vi "Simple TCP Test.vi"() -> ()   [LabVIEW 2020, in "VectoScratch.lvlib"]
uses:
  VectoScratch.lvlib
  Vecto/TCPMessaging/TCPMessaging.lvclass
  Simple TCP Handler/Simple TCP Handler.lvclass
  Vecto/TCPMessageService/TCPMessageAPI.lvclass
  Vecto/proto/TcpClientHello/Data.ctl
  Vecto/proto/TcpClientHello/TcpClientHello.lvlib
  Vecto/SequenceCountService/SequenceCountService.lvclass
  C:/dev/lv20CE/relink/lv-vecto/Vecto/TCPConnectionHandler/TCPConnectionHandler.lvclass
  C:/dev/lv20CE/relink/lv-vecto/Vecto/TCPMessageHandler/TCPMessageHandler.lvclass
  Vecto/Connection State.ctl
  Vecto/Vecto.lvlib
panel:
  out "Server Read":i32
  out "Client Read":i32
  out "Server Send":i32
  in  "Server Stop":bool
  in  "Client Stop":bool
  out "Client Send":i32
  out "Server Error":errorcluster
  out "Client Error":errorcluster
  out "Server State":T1=enum."Disconnected"
  out "Client State":T1=enum."Disconnected"
  # "Server send counts at ~half the speed of the client."
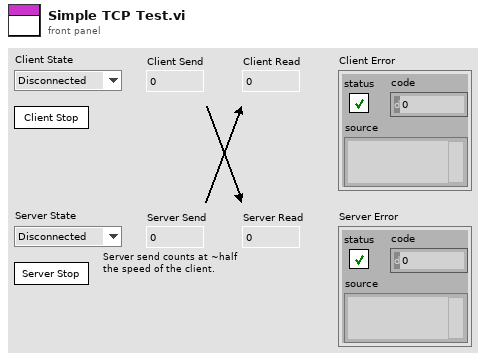
[diagram p1: front panel]
types:
  T1 = typedef "Vecto.lvlib/Connection State.ctl" = enum16{"Connected", "Disconnected"}
  T2 = typedef "TcpClientHello.lvlib/Data.ctl" = cluster{"node_id":u32, "system":string, "cluster":string, "node_name":string, "app_version":string, "config_version":string, "config_hash":string}
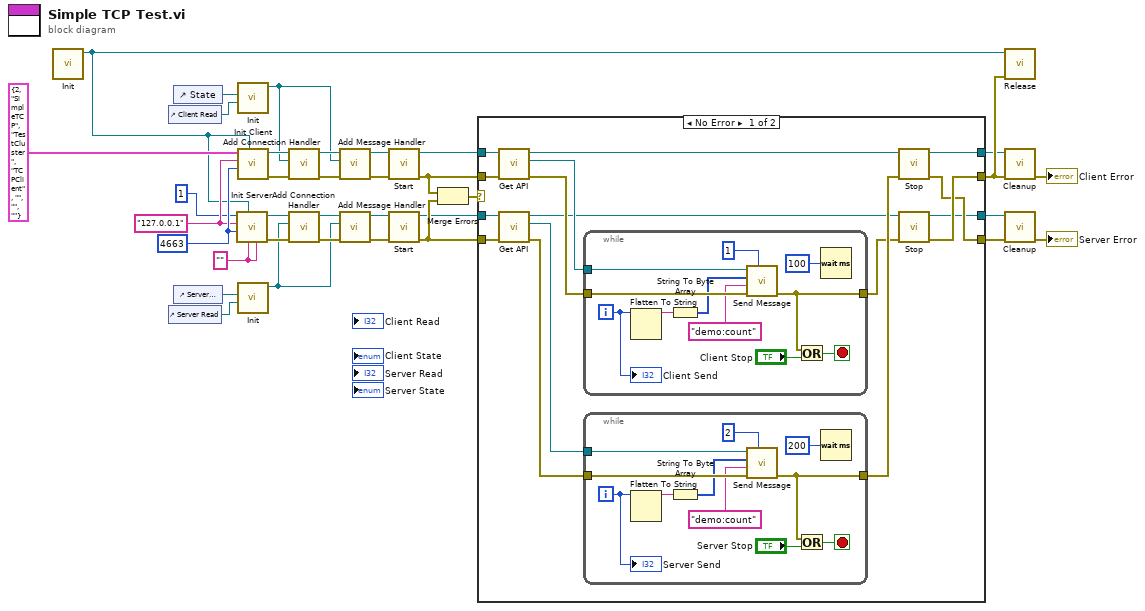
[diagram p0: block diagram]
diagram:
  w1 = "" ("Local Config Version")
  w34 = u16 4663 ("Bind Port")
  w33 = "127.0.0.1" ("Bind Address")
  n1 = call "Init.vi"() -> ("SequenceCountService out"=w2:refnum<class "SequenceCountService.lvclass">)  [unwired: 10 in, 1 out]
  n2 = control-ref of="Client Read"() -> (w5:refnum<vi>)
  n3 = control-ref of="Server Read"() -> (w6:refnum<vi>)
  n4 = control-ref of="State"() -> (w31:refnum<vi>)
  n5 = control-ref of="Server State"() -> (w23:refnum<vi>)
  n6 = call "Init Server.vi"("Local Config Hash"=w1, "Local Config Version"=w1, "SequenceCountService"=w2, "Bind Port"=w34, "Bind Address"=w33, "Node ID"=u32 1) -> ("error out"=w17:errorcluster, "TCPMessaging out"=w18:refnum<class "TCPMessaging.lvclass">)  [unwired: 4 in]
  n7 = call "Init.vi"("Value"=w5, "State"=w31) -> ("Simple TCP Handler out"=w27:refnum<class "Simple TCP Handler.lvclass">)  [unwired: 8 in, 1 out]
  n8 = call "Init Client.vi"("SequenceCountService"=w2, "Remote Port"=w34, "Remote Address"=w33, "Client Info"=T2 {"node_id"=2, "system"="SimpleTCP", "cluster"="TestCluster", "node_name"="TCPClient", "app_version"="", "config_version"="", "config_hash"=""}) -> ("error out"=w29:errorcluster, "TCPMessaging out"=w30:refnum<class "TCPMessaging.lvclass">)  [unwired: 6 in]
  n9 = call "Init.vi"("Value"=w6, "State"=w23) -> ("Simple TCP Handler out"=w4:refnum<class "Simple TCP Handler.lvclass">)  [unwired: 8 in, 1 out]
  n10 = call "Add Connection Handler.vi"("error in (no error)"=w29, "TCPConnectionHandler"=w27, "TCPMessaging in"=w30) -> ("error out"=w26:errorcluster, "TCPMessaging out"=w28:refnum<class "TCPMessaging.lvclass">)  [unwired: 7 in]
  n11 = call "Add Connection Handler.vi"("error in (no error)"=w17, "TCPConnectionHandler"=w4, "TCPMessaging in"=w18) -> ("error out"=w20:errorcluster, "TCPMessaging out"=w19:refnum<class "TCPMessaging.lvclass">)  [unwired: 7 in]
  n12 = call "Add Message Handler.vi"("error in (no error)"=w26, "TCPMessageHandler"=w27, "TCPMessaging in"=w28) -> ("error out"=w24:errorcluster, "TCPMessaging out"=w25:refnum<class "TCPMessaging.lvclass">)  [unwired: 7 in]
  n13 = call "Add Message Handler.vi"("error in (no error)"=w20, "TCPMessageHandler"=w4, "TCPMessaging in"=w19) -> ("error out"=w22:errorcluster, "TCPMessaging out"=w21:refnum<class "TCPMessaging.lvclass">)  [unwired: 7 in]
  n14 = call "Start.vi"("error in (no error)"=w24, "TCPMessaging in"=w25) -> ("error out"=w15:errorcluster, "TCPMessaging out"=w12:refnum<class "TCPMessaging.lvclass">)  [unwired: 8 in]
  n15 = call "Start.vi"("error in (no error)"=w22, "TCPMessaging in"=w21) -> ("error out"=w14:errorcluster, "TCPMessaging out"=w13:refnum<class "TCPMessaging.lvclass">)  [unwired: 8 in]
  n16 = Merge Errors(w15, w14) -> (w16:errorcluster)
  n17 = case shown="No Error" w16 {
    tunnel: w15 -> [w49 w77]
    tunnel: w14 -> [w47 w76]
    tunnel: w13 -> [w48 w75]
    tunnel: w12 -> [w50 w74]
    tunnel: [w41 w77] -> w35
    tunnel: [w39 w76] -> w9
    tunnel: [w38 w75] -> w10
    tunnel: [w40 w74] -> w11
    frame No Error {
      n18 = call "Get API.vi"("error in (no error)"=w49, "TCPMessaging in"=w50) -> ("error out"=w45:errorcluster, "TCP Messaging API"=w46:refnum<class "TCPMessageAPI.lvclass">, "TCPMessaging out"=w42:refnum<class "TCPMessaging.lvclass">)  [unwired: 7 in]
      n19 = call "Get API.vi"("error in (no error)"=w47, "TCPMessaging in"=w48) -> ("error out"=w36:errorcluster, "TCP Messaging API"=w37:refnum<class "TCPMessageAPI.lvclass">, "TCPMessaging out"=w44:refnum<class "TCPMessaging.lvclass">)  [unwired: 7 in]
      n20 = while {
        tunnel: w46 -> [w73]
        tunnel: w45 -> [w71]
        tunnel: [w64] -> w43
        i -> [w68]
        stop <- w65 stop-if-true
        n21 = Flatten To String(anything=w68) -> (data string=w70:string)  [unwired: 3 in, 2 out]
        n22 = String To Byte Array(string=w70) -> (unsigned byte array=w69:u8[])
        n23 = call "Send Message.vi"("Target ID"=u32 1 ("Target Node"), "error in (no error)"=w71, "Type"="demo:count", "Payload"=w69, "TCPMessageService in"=w73) -> ("error out"=w64:errorcluster)  [unwired: 5 in, 1 out]
        n24 = Or(x=w64, y="Client Stop") -> (x .or. y?=w65:bool)
        n25 = Wait (ms)(milliseconds to wait=u32 100) -> ()  [unwired: 1 out]
        "Client Send" <- w68
      }
      n26 = while {
        tunnel: w37 -> [w62]
        tunnel: w36 -> [w60]
        tunnel: [w53] -> w51
        i -> [w57]
        stop <- w54 stop-if-true
        n27 = Flatten To String(anything=w57) -> (data string=w59:string)  [unwired: 3 in, 2 out]
        n28 = String To Byte Array(string=w59) -> (unsigned byte array=w58:u8[])
        n29 = call "Send Message.vi"("Target ID"=u32 2 ("Target Node"), "error in (no error)"=w60, "Type"="demo:count", "Payload"=w58, "TCPMessageService in"=w62) -> ("error out"=w53:errorcluster)  [unwired: 5 in, 1 out]
        n30 = Or(x=w53, y="Server Stop") -> (x .or. y?=w54:bool)
        n31 = Wait (ms)(milliseconds to wait=u32 200) -> ()  [unwired: 1 out]
        "Server Send" <- w57
      }
      n32 = call "Stop.vi"("error in (no error)"=w51, "TCPMessaging in"=w42) -> ("error out"=w39:errorcluster, "TCPMessaging out"=w40:refnum<class "TCPMessaging.lvclass">)  [unwired: 8 in]
      n33 = call "Stop.vi"("error in (no error)"=w43, "TCPMessaging in"=w44) -> ("error out"=w41:errorcluster, "TCPMessaging out"=w38:refnum<class "TCPMessaging.lvclass">)  [unwired: 8 in]
    }
    frame Error {
    }
  }
  n34 = call "Release.vi"("error in (no error)"=w35, "SequenceCountService in"=w2) -> ()  [unwired: 9 in, 1 out]
  n35 = call "Cleanup.vi"("error in (no error)"=w35, "TCPMessaging in"=w11) -> ("error out"=→"Client Error":errorcluster)  [unwired: 9 in]
  n36 = call "Cleanup.vi"("error in (no error)"=w9, "TCPMessaging in"=w10) -> ("error out"=→"Server Error":errorcluster)  [unwired: 9 in]
